vi "Read Roles.vi"(8 "error in (no error)":errorcluster, 11 "NormalDefensiveWithDuelistPlay in":refnum<class "NormalDefensiveWithDuelistPlay.lvclass">) -> (0 "error out":errorcluster, 2 "Roles":T1, 3 "NormalDefensiveWithDuelistPlay out":refnum<class "NormalDefensiveWithDuelistPlay.lvclass">)   [LabVIEW 2023, in "NormalDefensiveWithDuelistPlay.lvclass"]
uses:
  NormalDefensiveWithDuelistPlay.lvclass
  DefenderAreaRole_class/DefenderAreaRole.lvclass
  DuelistRole_class/DuelistRole.lvclass
  NormalDefensiveWithDuelistPlay.lvclass/NormalDefensiveWithDuelistPlay.ctl
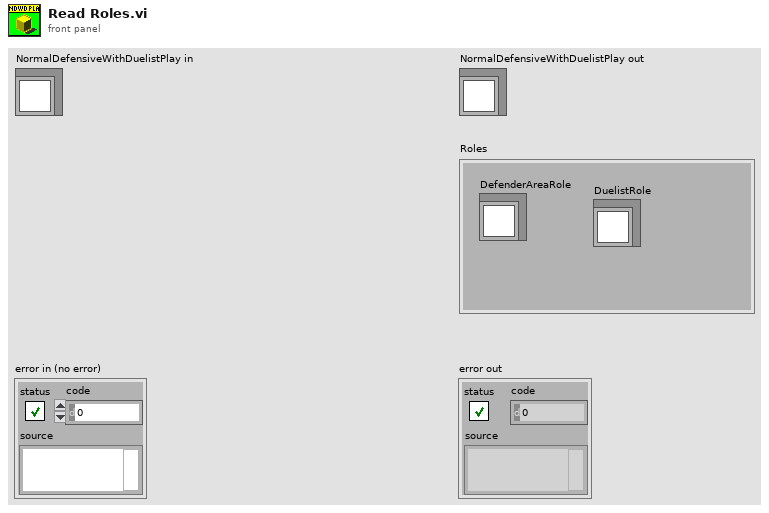
[diagram p1: front panel]
types:
  T1 = cluster{"DefenderAreaRole":refnum<class "DefenderAreaRole.lvclass">, "DuelistRole":refnum<class "DuelistRole.lvclass">}
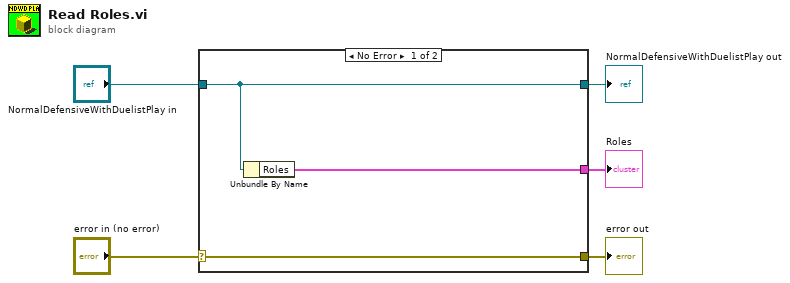
[diagram p0: block diagram]
diagram:
  n1 = case shown="No Error" "error in (no error)" {
    selector: "error in (no error)" -> [w8 w9]
    tunnel: [w8 w9] -> w4
    tunnel: [w7 w10] -> w2
    tunnel: "NormalDefensiveWithDuelistPlay in" -> [w7 w10]
    tunnel: [w6 _] -> w1
    frame No Error {
      n2 = Unbundle By Name(w7) -> ("Roles"=w6:T1)
    }
    frame Error {
    }
  }
  "error out" <- w4
  "NormalDefensiveWithDuelistPlay out" <- w2
  "Roles" <- w1
